vi "ColumbiaSonicare.vi"() -> ()   [LabVIEW 2022 SP3]
uses:
  Doppler data processing/Doppler/dopplerV6.llb/AI Waveform Scan (waveform).vi
  <vilib>/sound/lvsound.llb/Sound Format.ctl
  Doppler data processing/Doppler/dopplerV6.llb/AI Read (waveform).vi
panel:
  out "Stop (F3)":bool
  in  "EKGs between exposures":i32=1 min=0 max=50
  in  "Time between exposures (s)":sgl=0.1 min=0 format="%.1f"
  out "Exp Count":i32
  in  "Number of Exposures":i32=1 min=1
  in  "Mode":enum32{"HIFU", "Thromb"}(tab)
  in  "Skip":bool
  in  "Therapy Duration (s)":dbl=0.1 min=0.1 max=10.0 step=0.1 format="%.1f"
  out "# of Bursts":i32=1 min=1
  out "Elapsed\nTime (s)":i32=1 min=1
  out "PRF time  (ms)":sgl format="%.3f"
  in  "exp per cycle  (ms)":sgl=0.5 format="%.3f"
  in  "Total  exp. \ntime  (s)":sgl=1.0 min=0.001 format="%.2f"
  out "PRF  (kHz)":sgl=1.0 min=0.001 format="%.3f"
  in  "Duty Cycle":sgl=0.5 min=0 max=1 format="%.2f"
  in  "EKG ?":bool=TRUE
  in  "Re-Zero Trig":bool
  out "waveform data":waveform(dbl)[](array[waveform])
  in  "New EKG (F1)":bool
  in  "Exit Program (F2)":bool
  out "EKG":waveform(dbl)[](graph)
  in  "Fire Therapy (ESC)":bool
  out "Therapy Delay (s)":dbl=1.0 format="%.3f"
  # "1. Select EKG mode with switch below.\n2. If in EKG mode, update EKG trace with New EKG (F1).\n2a. Choose to have EKGs or fixed time interval between exposures.\n3. Drag pink line to mark start time of exposure and trigger level.\n4. Set time duration of exposure (0.1 s steps).\n5. Choose number of exposures and time between exposures (0.1 s min in EKG mode).\n6. Start exposure with Fire Therapy (ESC).\n7. Press pop up Stop Exp for emergency stop.\n8. To exit program, Press Exit Program (F2) to  terminate program.\n9. Thromb tab permits exposures of a fixed PRF, duty cycle, and time duration."
  # "© 2003 Riverside Research Institute"
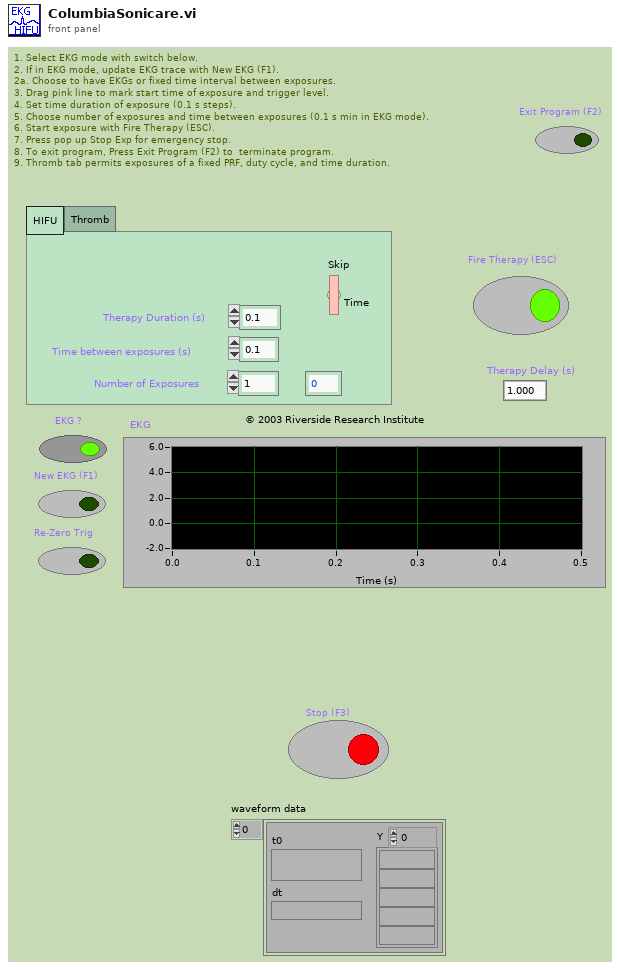
[diagram p1: front panel]
types:
  T1 = cluster{"coupling (no change:0)":enum16{"no change", "DC", "AC", "GND", "internal ref."}, "input config (no change:0)":u16}[]
  T2 = cluster{"high limit (0.0)":sgl, "low limit (0.0)":sgl}[]
  T3 = cluster{"trigger type (no trig:0)":enum16{"no trigger", "analog", "digital A", "digital B", "scan clock gate", "software analog "}, "pretrigger scans (0)":i32, "edge or slope \n(no change)":enum16{"no change", "rising", "falling"}, "analog chan (-) & level (0.0)":cluster{"trigger channel (empty)":string, "level (0.0)":sgl}, "scan clock source\n(no change:0)":enum16{"no change", "internal", "I/O Connector", "RTSI"}}
  T4 = typedef "Sound Format.ctl" = cluster{"sound quality":enum16{"mono", "stereo"}, "rate":enum16{"11025", "22050", "44100", "8000"}, "bits per sample":enum16{"8 bit", "16 bit"}}
  T5 = enum16{"no trigger", "analog", "digital A", "digital A & B", "scan clock gate"}
  T6 = cluster{"trigger channel (empty)":string, "Cursor.Cursor Y":dbl}
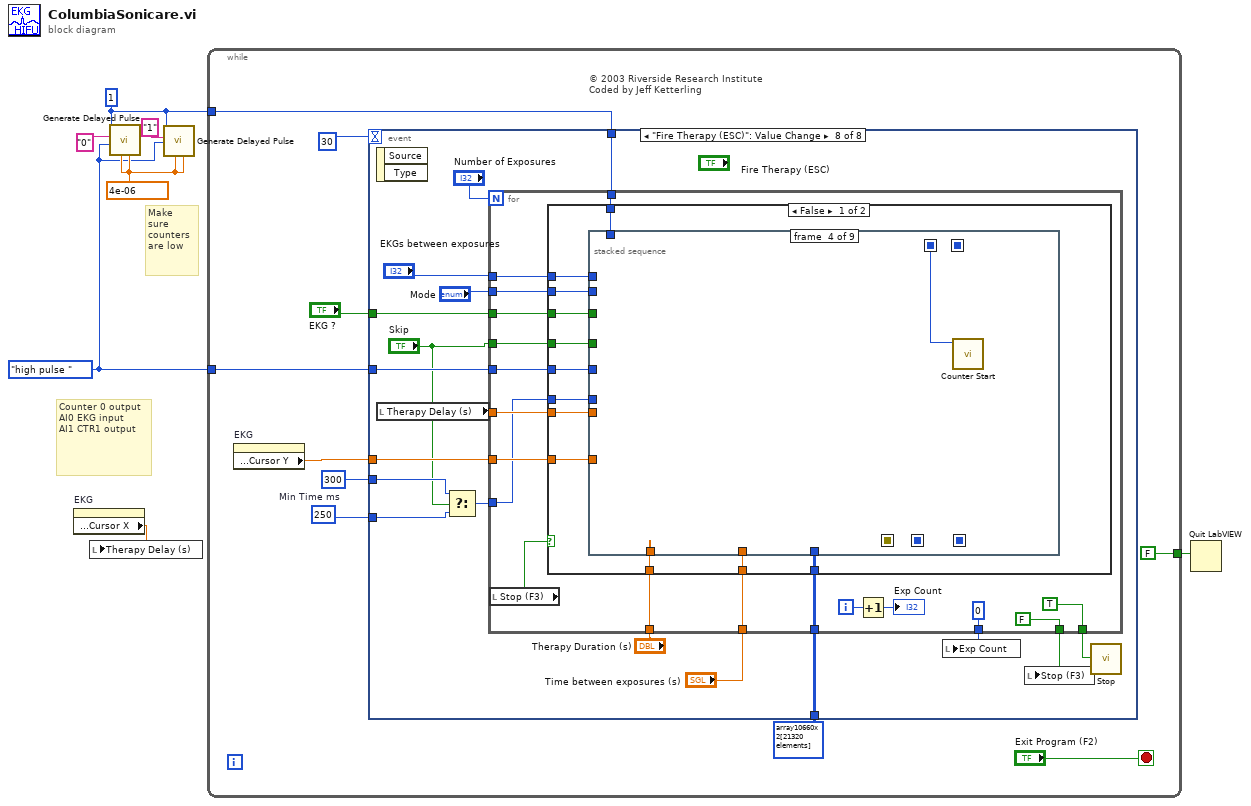
[diagram p0: block diagram]
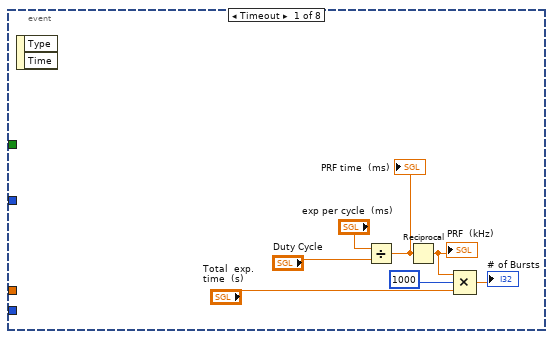
[diagram p2: hidden frame]
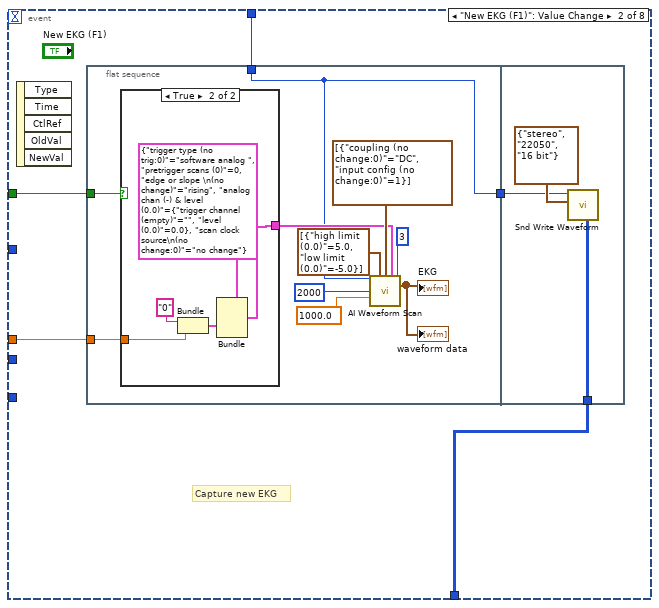
[diagram p3: hidden frame]
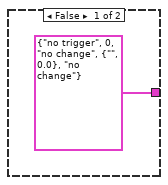
[diagram p4: hidden frame]
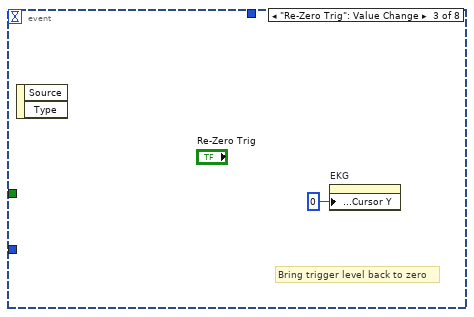
[diagram p5: hidden frame]
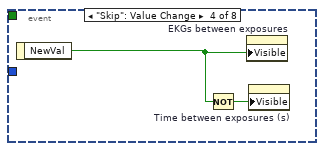
[diagram p6: hidden frame]
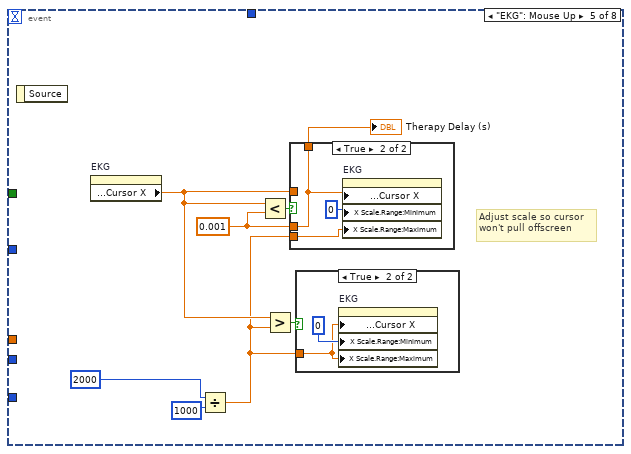
[diagram p7: hidden frame]
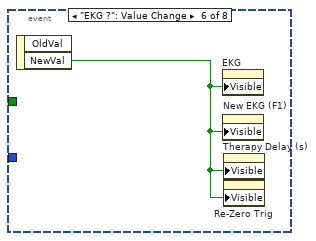
[diagram p10: hidden frame]
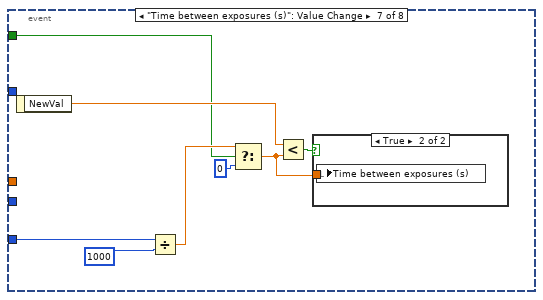
[diagram p11: hidden frame]
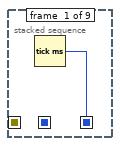
[diagram p13: hidden frame]
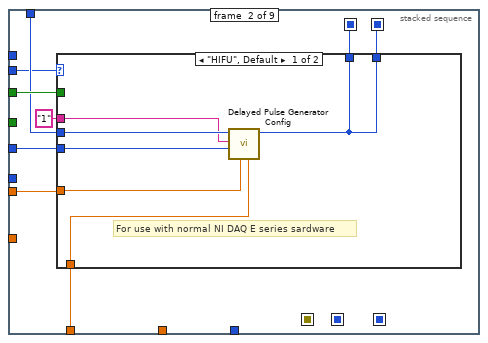
[diagram p14: hidden frame]
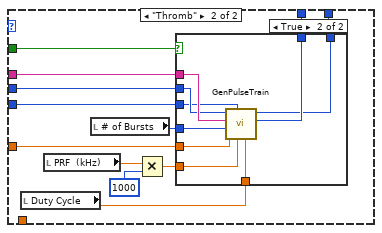
[diagram p15: hidden frame]
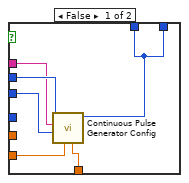
[diagram p16: hidden frame]
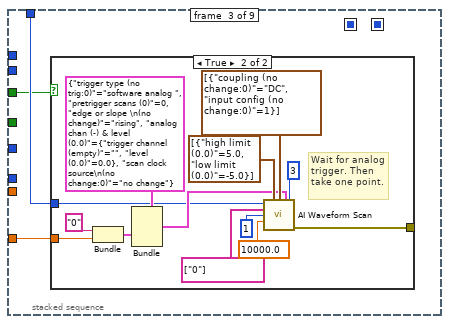
[diagram p17: hidden frame]
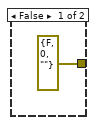
[diagram p18: hidden frame]
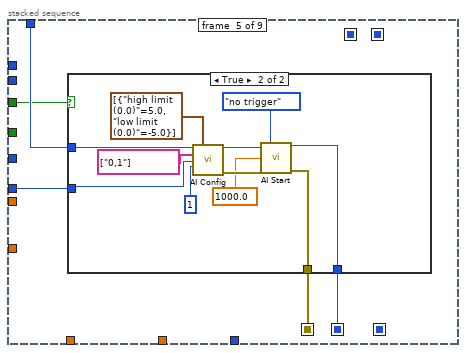
[diagram p19: hidden frame]
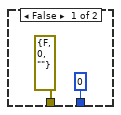
[diagram p20: hidden frame]
diagram:
  w2 = enum16{"high pulse ", "low pulse"}."high pulse " ("pulse polarity (high:0)")
  w3 = 4e-06
  w5 = 1
  # "Counter 0 output\nAI0 EKG input\nAI1 CTR1 output"
  # "Make sure counters are low"
  n1 = property on="EKG" class="WFGraph (strict)"() -> ("Cursor.Cursor Position:Cursor X"=w1:dbl)  [unwired: 2 in, 2 out]
  n2 = local write "Therapy Delay (s)"(w1) -> ()
  n3 = call <vilib>:"Generate Delayed Pulse.vi"("pulse width (s or cycles)"=w3, "pulse delay (s or cycles)"=w3, "pulse polarity (high:0)"=w2, "counter"="0", "device"=w5) -> ()  [unwired: 4 in, 3 out]
  n4 = call <vilib>:"Generate Delayed Pulse.vi"("pulse width (s or cycles)"=w3, "pulse delay (s or cycles)"=w3, "pulse polarity (high:0)"=w2, "counter"="1", "device"=w5) -> ()  [unwired: 4 in, 3 out]
  n5 = while {
    tunnel: w5 -> [w16]
    tunnel: [FALSE] -> w7
    tunnel: w2 -> [w13]
    stop <- "Exit Program (F2)" stop-if-true
    w12 = 250  # Min Time ms
    # "© 2003 Riverside Research Institute\nCoded by Jeff Ketterling"
    n6 = property on="EKG" class="WFGraph (strict)"() -> ("Cursor.Cursor Position:Cursor Y"=w8:dbl)  [unwired: 2 in, 2 out]
    n7 = event shown="[7] \"Fire Therapy (ESC)\": Value Change" {
      selector: _ -> [_ _ _ _ _ _ _ _]
      dyn-events: _ -> [_ _ _ _ _ _ _ _]
      timeout: 30 -> [_ _ _ _ _ _ _ _]
      tunnel: w16 -> [_ w29 _ _ _ _ _ w88]
      tunnel: w8 -> [_ w28 _ _ _ _ _ w86]
      tunnel: i16[][] array10660x2[21320 elements] ("stereo 16-bit") -> [_ w27 _ _ _ _ _ w87]
      tunnel: "EKG ?" -> [_ w26 _ _ _ _ w67 w91]
      tunnel: w12 -> [_ _ _ _ _ _ w68 w79]
      tunnel: w13 -> [_ _ _ _ _ _ _ w90]
      tunnel: 300 -> [_ _ _ _ _ _ _ w81]
      event Timeout {
        n8 = event-data() -> ()  [unwired: 1 in, 2 out]
        n9 = Divide(x="exp per cycle  (ms)", y="Duty Cycle") -> (x/y=w23:sgl)
        "PRF time  (ms)" <- w23
        n10 = Reciprocal(x=w23) -> (1/x=w22:sgl)
        "PRF  (kHz)" <- w22
        n11 = Compound Arithmetic op=MULTIPLY(w22, 1000, "Total  exp. \ntime  (s)") -> (→"# of Bursts":sgl)
      }
      event "New EKG (F1)": Value Change {
        # "Capture new EKG"
        n12 = event-data() -> ()  [unwired: 1 in, 5 out]
        n13 = flat-sequence {
          tunnel: w26 -> [w32]
          tunnel: w29 -> [w30]
          tunnel: w28 -> [w31]
          tunnel: [w30] -> w25
          tunnel: w27 -> [w46]
          tunnel: w25 -> [w47]
          frame #0 {
            n14 = case shown="True" w32 {
              tunnel: [T3 {"trigger type (no trig:0)"=enum."no trigger", "pretrigger scans (0)"=0, "edge or slope \n(no change)"=enum."no change", "analog chan (-) & level (0.0)"={"trigger channel (empty)"="", "level (0.0)"=0.0}, "scan clock source\n(no change:0)"=enum."no change"} ("trigger and clock (no trig, int clk)") w45] -> w34
              tunnel: w31 -> [_ w44]
              frame False {
              }
              frame True {
                n15 = Bundle("trigger channel (empty)"="0", "Cursor.Cursor Y"=w44) -> (w42:T6)  [unwired: 1 in]
                n16 = Bundle(cluster=T3 {"trigger type (no trig:0)"=enum."software analog ", "pretrigger scans (0)"=0, "edge or slope \n(no change)"=enum."rising", "analog chan (-) & level (0.0)"={"trigger channel (empty)"="", "level (0.0)"=0.0}, "scan clock source\n(no change:0)"=enum."no change"} ("trigger and clock (no trig, int clk)"), "analog chan (-) & level (0.0)"=w42) -> (w45:T3)  [unwired: 4 in]
              }
            }
            n17 = call-poly "AI Waveform Scan.vi"("device (1)"=w30, "input limits (no change)"=T2 [{"high limit (0.0)"=5.0, "low limit (0.0)"=-5.0}], "coupling & input config (no change:0)"=T1 [{"coupling (no change:0)"=enum."DC", "input config (no change:0)"=1}], "trigger and clock (no trig, int clk)"=w34, "time limit in sec \n(computed:-1)"=3, "number of scans\n(1000)"=2000, "scan rate (1000 scans/sec)"=sgl 1000.0) -> ("waveform data"=→"EKG" →"waveform data":waveform(dbl)[])  [unwired: 7 in, 1 out]
          }
          frame #1 {
            n18 = call <vilib>:"Snd Write Waveform.vi"("stereo 16-bit"=w46, "sound format"=T4 {"sound quality"=enum."stereo", "rate"=enum."22050", "bits per sample"=enum."16 bit"}, "device (0)"=w47) -> ()  [unwired: 8 in, 1 out]
          }
        }
      }
      event "Re-Zero Trig": Value Change {
        # "Bring trigger level back to zero"
        n19 = event-data() -> ()  [unwired: 1 in, 2 out]
        n20 = property on="EKG" class="WFGraph (strict)"("Cursor.Cursor Position:Cursor Y"=0) -> ()  [unwired: 2 in, 2 out]
      }
      event "Skip": Value Change {
        n21 = event-data() -> ("NewVal"=w51:bool)  [unwired: 1 in]
        n22 = Not(x=w51) -> (.not. x?=w50:bool)
        n23 = property on="EKGs between exposures" class="DigNum (strict)"("Visible"=w51) -> ()  [unwired: 2 in, 2 out]
        n24 = property on="Time between exposures (s)" class="DigNum (strict)"("Visible"=w50) -> ()  [unwired: 2 in, 2 out]
      }
      event "EKG": Mouse Up {
        w58 = 0.001
        # "Adjust scale so cursor won't pull offscreen"
        n25 = event-data() -> ()  [unwired: 1 in, 1 out]
        n26 = property on="EKG" class="WFGraph (strict)"() -> ("Cursor.Cursor Position:Cursor X"=w55:dbl)  [unwired: 2 in, 2 out]
        n27 = Divide(x=2000, y=1000) -> (x/y=w53:dbl)
        n28 = Less?(x=w55, y=w58) -> (x < y?=w59:bool)
        n29 = Greater?(x=w55, y=w53) -> (0:w57:bool)
        n30 = case shown="True" w59 {
          tunnel: w55 -> [w62 _]
          tunnel: [w62 w65] -> w56
          tunnel: w58 -> [_ w65]
          tunnel: w53 -> [_ w63]
          frame False {
          }
          frame True {
            n31 = property on="EKG" class="WFGraph (strict)"("Cursor.Cursor Position:Cursor X"=w65, "X Scale.Range:Minimum"=0, "X Scale.Range:Maximum"=w63) -> ()  [unwired: 2 in, 2 out]
          }
        }
        "Therapy Delay (s)" <- w56
        n32 = case shown="True" w57 {
          tunnel: w53 -> [_ w60]
          frame False {
          }
          frame True {
            n33 = property on="EKG" class="WFGraph (strict)"("Cursor.Cursor Position:Cursor X"=w60, "X Scale.Range:Minimum"=0, "X Scale.Range:Maximum"=w60) -> ()  [unwired: 2 in, 2 out]
          }
        }
      }
      event "EKG ?": Value Change {
        n34 = event-data() -> ("NewVal"=w66:bool)  [unwired: 1 in, 1 out]
        n35 = property on="EKG" class="WFGraph (strict)"("Visible"=w66) -> ()  [unwired: 2 in, 2 out]
        n36 = property on="New EKG (F1)" class="Bool"("Visible"=w66) -> ()  [unwired: 2 in, 2 out]
        n37 = property on="Therapy Delay (s)" class="DigNum (strict)"("Visible"=w66) -> ()  [unwired: 2 in, 2 out]
        n38 = property on="Re-Zero Trig" class="Bool"("Visible"=w66) -> ()  [unwired: 2 in, 2 out]
      }
      event "Time between exposures (s)": Value Change {
        n39 = event-data() -> ("NewVal"=w69:sgl)  [unwired: 1 in]
        n40 = Divide(x=w68, y=1000) -> (x/y=w70:dbl)
        n41 = Select(t=w70, s=w67, f=0) -> (s? t:f=w72:dbl)
        n42 = Less?(x=w69, y=w72) -> (x < y?=w73:bool)
        n43 = case shown="True" w73 {
          tunnel: w72 -> [_ w75]
          frame False {
          }
          frame True {
            n44 = local write "Time between exposures (s)"(w75) -> ()
          }
        }
      }
      event "Fire Therapy (ESC)": Value Change {
        n45 = event-data() -> ()  [unwired: 1 in, 2 out]
        n46 = local read "Therapy Delay (s)"() -> (w89:dbl)
        n47 = Select(t=w81, s="Skip", f=w79) -> (s? t:f=w78:i32)
        n48 = for {
          N: "Number of Exposures" -> [_]
          tunnel: w88 -> [w111]
          tunnel: w91 -> [w110]
          tunnel: w86 -> [w109]
          tunnel: w87 -> [w108]
          tunnel: "Time between exposures (s)" -> [w106]
          tunnel: "Therapy Duration (s)" -> [w105]
          tunnel: "Mode" -> [w103]
          tunnel: w90 -> [w102]
          tunnel: w89 -> [w101]
          tunnel: "EKGs between exposures" -> [w100]
          tunnel: "Skip" -> [w99]
          tunnel: [0] -> w84
          tunnel: w78 -> [w97]
          tunnel: [TRUE] -> w77
          tunnel: [FALSE] -> w76
          i -> [w107]
          n49 = local read "Stop (F3)"() -> (w96:bool)
          n50 = case shown="False" w96 {
            tunnel: w111 -> [w123 _]
            tunnel: w110 -> [w122 _]
            tunnel: w109 -> [w121 _]
            tunnel: w108 -> [w120 _]
            tunnel: w106 -> [w119 _]
            tunnel: w105 -> [w118 _]
            tunnel: w103 -> [w117 _]
            tunnel: w102 -> [w116 _]
            tunnel: w97 -> [w115 _]
            tunnel: w101 -> [w114 _]
            tunnel: w100 -> [w113 _]
            tunnel: w99 -> [w112 _]
            frame False {
              n51 = stacked-sequence {
                seq-local: [_ w131 _ _ _ _ _ _ _] -> [_ _ _ w184 _ w212 _ _ _]
                seq-local: [_ _ _ _ w188 _ _ _ _] -> [_ _ _ _ _ _ w232 _ _]
                seq-local: [_ _ _ _ w187 _ _ _ _] -> [_ _ _ _ _ _ w231 _ _]
                seq-local: [_ w127 _ _ _ _ _ _ _] -> [_ _ _ _ _ w206 _ _ _]
                seq-local: [w124 _ _ _ _ _ _ _ _] -> [_ _ _ _ _ _ _ _ w247]
                tunnel: w123 -> [_ w130 w169 _ w189 _ _ w239 w244]
                tunnel: w118 -> [_ w133 _ _ _ w209 _ _ _]
                tunnel: w122 -> [_ w132 w168 _ w185 _ w229 _ _]
                tunnel: w121 -> [_ _ w167 _ _ _ _ _ w243]
                tunnel: w120 -> [_ _ _ _ _ _ _ w240 _]
                tunnel: w119 -> [_ _ _ _ _ _ _ _ w246]
                tunnel: w117 -> [_ w129 _ _ _ w210 _ _ _]
                tunnel: w116 -> [_ w128 _ _ _ _ _ _ _]
                tunnel: w115 -> [_ _ _ _ w186 _ w230 _ _]
                tunnel: w114 -> [_ w125 _ _ _ w204 _ _ _]
                tunnel: w113 -> [_ _ _ _ _ _ _ _ w245]
                tunnel: w112 -> [_ _ _ _ _ _ _ _ w242]
                frame #0 {
                  n52 = Tick Count (ms)() -> (millisecond timer value=w124:u32)
                }
                frame #1 {
                  n53 = case shown="\"HIFU\", Default" w129 {
                    tunnel: w125 -> [w139 w143]
                    tunnel: w133 -> [w138 _]
                    tunnel: w132 -> [_ w144]
                    tunnel: [w135 w147] -> w131
                    tunnel: w130 -> [w137 w151]
                    tunnel: w128 -> [w136 w148]
                    tunnel: [w135 w142] -> w127
                    tunnel: "1" ("counter") -> [w134 w141]
                    frame "HIFU", Default {
                      # "For use with normal NI DAQ E series sardware"
                      n54 = call <vilib>:"Delayed Pulse Generator Config.vi"("pulse width (s or cycles)"=w138, "pulse delay (s or cycles)"=w139, "pulse polarity (high:0)"=w136, "counter"=w134, "device"=w137) -> ("taskID"=w135:u32)  [unwired: 3 in, 3 out]
                    }
                    frame "Thromb" {
                      n55 = local read "Duty Cycle"() -> (w140:sgl)
                      n56 = local read "PRF  (kHz)"() -> (w149:sgl)
                      n57 = local read "# of Bursts"() -> (w146:i32)
                      n58 = Multiply(x=w149, y=1000) -> (x*y=w145:sgl)
                      n59 = case shown="True" w144 {
                        tunnel: w151 -> [w157 w163]
                        tunnel: w140 -> [w156 w161]
                        tunnel: w145 -> [w155 w165]
                        tunnel: w148 -> [w154 w162]
                        tunnel: [w152 w160] -> w147
                        tunnel: w141 -> [w153 w166]
                        tunnel: w146 -> [_ w164]
                        tunnel: w143 -> [_ w159]
                        tunnel: [w152 w158] -> w142
                        frame False {
                          n60 = call <vilib>:"Continuous Pulse Generator Config.vi"("duty cycle (0.5)"=w156, "frequency (Hz)"=w155, "pulse polarity (high:0)"=w154, "counter"=w153, "device"=w157) -> ("taskID"=w152:u32)  [unwired: 3 in, 3 out]
                        }
                        frame True {
                          n61 = call "GenPulseTrain.vi"("duty cycle (0.5)"=w161, "frequency (Hz)"=w165, "pulse polarity (high:0)"=w162, "delay"=w159, "number of pulses (cont:0)"=w164, "counter"=w166, "device"=w163) -> ("[taskID of counter-1]"=w160:u32, "[taskID of counter]"=w158:u32)  [unwired: 2 in, 1 out]
                        }
                      }
                    }
                  }
                }
                frame #2 {
                  n62 = case shown="True" w168 {
                    tunnel: w169 -> [_ w173]
                    tunnel: w167 -> [_ w174]
                    tunnel: [errorcluster {"status"=FALSE, "code"=0, "source"=""} ("error out") w171] -> _
                    frame False {
                    }
                    frame True {
                      # "Wait for analog trigger. Then take one point."
                      n63 = Bundle("trigger channel (empty)"="0", "Cursor.Cursor Y"=w174) -> (w175:T6)  [unwired: 1 in]
                      n64 = Bundle(cluster=T3 {"trigger type (no trig:0)"=enum."software analog ", "pretrigger scans (0)"=0, "edge or slope \n(no change)"=enum."rising", "analog chan (-) & level (0.0)"={"trigger channel (empty)"="", "level (0.0)"=0.0}, "scan clock source\n(no change:0)"=enum."no change"} ("trigger and clock (no trig, int clk)"), "analog chan (-) & level (0.0)"=w175) -> (w177:T3)  [unwired: 4 in]
                      n65 = call-poly "AI Waveform Scan.vi"("device (1)"=w173, "input limits (no change)"=T2 [{"high limit (0.0)"=5.0, "low limit (0.0)"=-5.0}], "coupling & input config (no change:0)"=T1 [{"coupling (no change:0)"=enum."DC", "input config (no change:0)"=1}], "trigger and clock (no trig, int clk)"=w177, "time limit in sec \n(computed:-1)"=3, "channels (0)"=tag[] ["0"], "number of scans\n(1000)"=1, "scan rate (1000 scans/sec)"=sgl 10000.0) -> ("error out"=w171:errorcluster)  [unwired: 6 in, 1 out]
                    }
                  }
                }
                frame #3 {
                  n66 = call <vilib>:"Counter Start.vi"("taskID"=w184) -> ()  [unwired: 9 in, 2 out]
                }
                frame #4 {
                  n67 = case shown="True" w185 {
                    tunnel: w189 -> [_ w195]
                    tunnel: [u32 0 ("taskID out") w194] -> w188
                    tunnel: [errorcluster {"status"=FALSE, "code"=0, "source"=""} ("error out") w193] -> w187
                    tunnel: w186 -> [_ w192]
                    frame False {
                    }
                    frame True {
                      n68 = call "AI Config.vi"("device (1)"=w195, "input limits (no change)"=T2 [{"high limit (0.0)"=5.0, "low limit (0.0)"=-5.0}], "channels (0)"=tag[] ["0,1"], "buffer size (1000 scans)"=w192, "[group] (0)"=1) -> ("taskID"=w197:u32, "error out"=w202:errorcluster)  [unwired: 8 in, 1 out]
                      n69 = call "AI Start.vi"("taskID in"=w197, "trigger type (no trig:0)"=T5."no trigger", "scan rate (1000 scans/sec)"=sgl 1000.0, "error in (no error)"=w202) -> ("taskID out"=w194:u32, "error out"=w193:errorcluster)  [unwired: 8 in, 2 out]
                    }
                  }
                }
                frame #5 {
                  n70 = local read "Total  exp. \ntime  (s)"() -> (w203:sgl)
                  n71 = Not Equal To 0?(x=w210) -> (x != 0?=w211:bool)
                  n72 = Select(t=w203, s=w211, f=w209) -> (s? t:f=w207:dbl)
                  n73 = Add(x=w204, y=w207) -> (x+y=w208:dbl)
                  n74 = Multiply(x=w208, y=1000) -> (x*y=w205:dbl)
                  n75 = Tick Count (ms)() -> (millisecond timer value=w214:u32)
                  n76 = while {
                    tunnel: w212 -> [w226]
                    tunnel: w214 -> [w224]
                    tunnel: w205 -> [w223]
                    tunnel: w206 -> [w217]
                    stop <- w221 stop-if-true
                    # "Stop if aborted or time limit up"
                    n77 = Tick Count (ms)() -> (millisecond timer value=w225:u32)
                    n78 = Subtract(x=w225, y=w224) -> (x-y=w220:u32)
                    n79 = call "Stop.vi"("Close FP"=FALSE) -> ("Stop Now?"=w215:bool)  [unwired: 1 in]
                    "Stop (F3)" <- w215
                    n80 = Greater?(x=w220, y=w223) -> (0:w222:bool)
                    n81 = Divide(x=w220, y=1000) -> (x/y=→"Elapsed\nTime (s)":dbl)
                    n82 = Or(x=w215, y=w222) -> (x .or. y?=w221:bool)
                    n83 = case shown="True" w221 {
                      tunnel: w226 -> [_ w228]
                      tunnel: w217 -> [_ w227]
                      frame False {
                      }
                      frame True {
                        n84 = call <vilib>:"Counter Stop.vi"("taskID"=w228) -> ()  [unwired: 5 in, 2 out]
                        n85 = call <vilib>:"Counter Stop.vi"("taskID"=w227) -> ()  [unwired: 5 in, 2 out]
                      }
                    }
                  }
                }
                frame #6 {
                  n86 = case shown="True" w229 {
                    tunnel: w232 -> [_ w235]
                    tunnel: w231 -> [_ w234]
                    tunnel: w230 -> [_ w233]
                    frame False {
                    }
                    frame True {
                      n87 = call-poly "AI Read.vi"("taskID in"=w235, "number of scans to read (-1:all)"=w233, "error in (no error)"=w234) -> ("taskID out"=w238:u32, "waveform data"=w236:waveform(dbl)[], "error out"=w237:errorcluster)  [unwired: 7 in, 3 out]
                      n88 = local write "EKG"(w236) -> ()
                      n89 = call "AI Clear.vi"("error in (no error)"=w237, "taskID in"=w238) -> ()  [unwired: 4 in, 2 out]
                    }
                  }
                }
                frame #7 {
                  n90 = call <vilib>:"Snd Write Waveform.vi"("stereo 16-bit"=w240, "sound format"=T4 {"sound quality"=enum."stereo", "rate"=enum."22050", "bits per sample"=enum."16 bit"}, "device (0)"=w239) -> ()  [unwired: 8 in, 1 out]
                }
                frame #8 {
                  n91 = case shown="True" w242 {
                    tunnel: w247 -> [w251 _]
                    tunnel: w246 -> [w248 _]
                    tunnel: w245 -> [_ w257]
                    tunnel: w244 -> [_ w256]
                    tunnel: w243 -> [_ w255]
                    frame False {
                      # "Wait remaining time."
                      # "Account for overhead times of earlier frames"
                      n92 = Tick Count (ms)() -> (millisecond timer value=w250:u32)
                      n93 = Multiply(x=w248, y=1000) -> (x*y=w253:sgl)
                      n94 = Subtract(x=w250, y=w251) -> (x-y=w249:u32)
                      n95 = Subtract(x=w253, y=w249) -> (x-y=w252:sgl)
                      n96 = Wait (ms)(milliseconds to wait=w252) -> ()  [unwired: 1 out]
                    }
                    frame True {
                      n97 = for {
                        N: w257 -> [_]
                        tunnel: w256 -> [w261]
                        tunnel: w255 -> [w260]
                        tunnel: [w259] -> _
                        # "Wait for analog trigger. Then take one point."
                        n98 = Bundle("trigger channel (empty)"="0", "Cursor.Cursor Y"=w260) -> (w263:T6)  [unwired: 1 in]
                        n99 = Bundle(cluster=T3 {"trigger type (no trig:0)"=enum."software analog ", "pretrigger scans (0)"=0, "edge or slope \n(no change)"=enum."rising", "analog chan (-) & level (0.0)"={"trigger channel (empty)"="", "level (0.0)"=0.0}, "scan clock source\n(no change:0)"=enum."no change"} ("trigger and clock (no trig, int clk)"), "analog chan (-) & level (0.0)"=w263) -> (w265:T3)  [unwired: 4 in]
                        n100 = call-poly "AI Waveform Scan.vi"("device (1)"=w261, "input limits (no change)"=T2 [{"high limit (0.0)"=5.0, "low limit (0.0)"=-5.0}], "coupling & input config (no change:0)"=T1 [{"coupling (no change:0)"=enum."DC", "input config (no change:0)"=1}], "trigger and clock (no trig, int clk)"=w265, "time limit in sec \n(computed:-1)"=3, "channels (0)"=tag[] ["0"], "number of scans\n(1000)"=2, "scan rate (1000 scans/sec)"=sgl 10000.0) -> ("error out"=w259:errorcluster)  [unwired: 6 in, 1 out]
                        n101 = Wait (ms)(milliseconds to wait=50) -> ()  [unwired: 1 out]
                      }
                    }
                  }
                }
              }
            }
            frame True {
            }
          }
          n102 = Increment(x=w107) -> (x+1=→"Exp Count":i32)
        }
        n103 = local write "Exp Count"(w84) -> ()
        n104 = local write "Stop (F3)"(w76) -> ()
        n105 = call "Stop.vi"("Close FP"=w77) -> ()  [unwired: 1 in, 1 out]
      }
    }
  }
  n106 = Quit LabVIEW(quit? (T)=w7) -> ()
